vi "Main.vi"() -> ()   [LabVIEW 2018] (continued)
                w3479 = u8 132 items=["I/O (P)"=128, "Input (I)"=129, "Output (Q)"=130, "Bit Memory (M)"=131, "Data (DB)"=132, "Instance Data (DI)"=133, "Local Data (L)"=134, "Predecessor Local Data (VL)"=135] ("寄存器类型")
                w3480 = u16 1 items=["byte", "word", "Dword"] ("数据类型")
                n2689 = local read "上一站号 (301)"() -> (w3472:string)
                n2690 = local read "上一站结果 (301)"() -> (w3471:string)
                n2691 = Decimal String To Number(string=w3472, default (0L)=u32 0 ("默认(0 I32)")) -> (number=w3489:u32)  [unwired: 1 in, 1 out]
                n2692 = call "S7_Write.vi"("TCP"=w3477, "寄存器类型"=w3479, "DB #"=u16 20, "写入地址"=u32 16, "数据类型"=w3480, "写入数据"=w3489, "error in"=w3476) -> ("TCP"=w3488:refnum<k5>, "error out"=w3487:errorcluster)  [unwired: 6 in, 1 out]
                n2693 = Equal?(x=w3471, y="OK") -> (x = y?=w3491:bool)
                n2694 = case shown="假" w3491 {
                  tunnel: [u32 2 ("写入数据") u32 1 ("写入数据")] -> w3492
                  frame False {
                  }
                  frame True {
                  }
                }
                n2695 = local read "扫码请求回复301"() -> (w3470:string)
                n2696 = call "S7_Write.vi"("TCP"=w3488, "寄存器类型"=w3485, "DB #"=u16 20, "写入地址"=u32 18, "数据类型"=w3484, "写入数据"=w3492, "error in"=w3487) -> ("TCP"=w3475:refnum<k5>, "error out"=w3474:errorcluster)  [unwired: 6 in, 1 out]
                n2697 = Decimal String To Number(string=w3470) -> (number=w3473:i32)  [unwired: 2 in, 1 out]
              }
            }
            n2698 = call "S7_Write.vi"("TCP"=w3395, "寄存器类型"=w3413, "DB #"=u16 20, "写入地址"=u32 4, "数据类型"=w3412, "写入数据"=w3393, "error in"=w3394) -> ("TCP"=w3388:refnum<k5>, "error out"=w3387:errorcluster)  [unwired: 6 in, 1 out]
            n2699 = case shown="真" "301数据回复输入" {
              tunnel: [999 w3466] -> w3386
              frame False {
              }
              frame True {
                n2700 = local read "数据保存请求回复301"() -> (w3465:string)
                n2701 = Decimal String To Number(string=w3465) -> (number=w3466:i32)  [unwired: 2 in, 1 out]
              }
            }
            n2702 = call "S7_Write.vi"("TCP"=w3388, "寄存器类型"=w3390, "DB #"=u16 20, "写入地址"=u32 6, "数据类型"=w3389, "写入数据"=w3386, "error in"=w3387) -> ("TCP"=w3385:refnum<k5>, "error out"=w3384:errorcluster)  [unwired: 6 in, 1 out]
            n2703 = case shown="真" "302扫码回复输入" {
              tunnel: [999 w3504] -> w3407
              tunnel: w3385 -> [w3499 w3518]
              tunnel: w3384 -> [w3498 w3517]
              tunnel: [w3499 w3506] -> w3406
              tunnel: [w3498 w3505] -> w3405
              frame False {
              }
              frame True {
                w3512 = u8 132 items=["I/O (P)"=128, "Input (I)"=129, "Output (Q)"=130, "Bit Memory (M)"=131, "Data (DB)"=132, "Instance Data (DI)"=133, "Local Data (L)"=134, "Predecessor Local Data (VL)"=135] ("寄存器类型")
                w3513 = u16 1 items=["byte", "word", "Dword"] ("数据类型")
                w3520 = u8 132 items=["I/O (P)"=128, "Input (I)"=129, "Output (Q)"=130, "Bit Memory (M)"=131, "Data (DB)"=132, "Instance Data (DI)"=133, "Local Data (L)"=134, "Predecessor Local Data (VL)"=135] ("寄存器类型")
                w3519 = u16 1 items=["byte", "word", "Dword"] ("数据类型")
                n2704 = local read "上一站号 (302)"() -> (w3503:string)
                n2705 = Decimal String To Number(string=w3503) -> (number=w3516:i32)  [unwired: 2 in, 1 out]
                n2706 = call "S7_Write.vi"("TCP"=w3518, "寄存器类型"=w3520, "DB #"=u16 20, "写入地址"=u32 20, "数据类型"=w3519, "写入数据"=w3516, "error in"=w3517) -> ("TCP"=w3508:refnum<k5>, "error out"=w3509:errorcluster)  [unwired: 6 in, 1 out]
                n2707 = local read "上一站结果 (302)"() -> (w3502:string)
                n2708 = local read "扫码请求回复302"() -> (w3501:string)
                n2709 = Equal?(x=w3502, y="OK") -> (x = y?=w3515:bool)
                n2710 = case shown="假" w3515 {
                  tunnel: [u32 2 ("写入数据") u32 1 ("写入数据")] -> w3507
                  frame False {
                  }
                  frame True {
                  }
                }
                n2711 = call "S7_Write.vi"("TCP"=w3508, "寄存器类型"=w3512, "DB #"=u16 20, "写入地址"=u32 22, "数据类型"=w3513, "写入数据"=w3507, "error in"=w3509) -> ("TCP"=w3506:refnum<k5>, "error out"=w3505:errorcluster)  [unwired: 6 in, 1 out]
                n2712 = Decimal String To Number(string=w3501) -> (number=w3504:i32)  [unwired: 2 in, 1 out]
              }
            }
            n2713 = call "S7_Write.vi"("TCP"=w3406, "寄存器类型"=w3410, "DB #"=u16 20, "写入地址"=u32 8, "数据类型"=w3411, "写入数据"=w3407, "error in"=w3405) -> ("TCP"=w3399:refnum<k5>, "error out"=w3400:errorcluster)  [unwired: 6 in, 1 out]
            n2714 = case shown="真" "302数据回复输入" {
              tunnel: [999 w3497] -> w3398
              frame False {
              }
              frame True {
                n2715 = local read "数据保存请求回复302"() -> (w3496:string)
                n2716 = Decimal String To Number(string=w3496) -> (number=w3497:i32)  [unwired: 2 in, 1 out]
              }
            }
            n2717 = call "S7_Write.vi"("TCP"=w3399, "寄存器类型"=w3403, "DB #"=u16 20, "写入地址"=u32 10, "数据类型"=w3404, "写入数据"=w3398, "error in"=w3400) -> ("TCP"=w3363:refnum<k5>, "error out"=w3362:errorcluster)  [unwired: 6 in, 1 out]
            n2718 = case shown="真" "303扫码回复输入" {
              tunnel: [999 w3443] -> w3368
              tunnel: w3363 -> [w3438 w3457]
              tunnel: w3362 -> [w3437 w3456]
              tunnel: [w3438 w3445] -> w3369
              tunnel: [w3437 w3444] -> w3370
              frame False {
              }
              frame True {
                w3451 = u8 132 items=["I/O (P)"=128, "Input (I)"=129, "Output (Q)"=130, "Bit Memory (M)"=131, "Data (DB)"=132, "Instance Data (DI)"=133, "Local Data (L)"=134, "Predecessor Local Data (VL)"=135] ("寄存器类型")
                w3452 = u16 1 items=["byte", "word", "Dword"] ("数据类型")
                w3459 = u8 132 items=["I/O (P)"=128, "Input (I)"=129, "Output (Q)"=130, "Bit Memory (M)"=131, "Data (DB)"=132, "Instance Data (DI)"=133, "Local Data (L)"=134, "Predecessor Local Data (VL)"=135] ("寄存器类型")
                w3458 = u16 1 items=["byte", "word", "Dword"] ("数据类型")
                n2719 = local read "上一站号 (303)"() -> (w3442:string)
                n2720 = Decimal String To Number(string=w3442) -> (number=w3455:i32)  [unwired: 2 in, 1 out]
                n2721 = call "S7_Write.vi"("TCP"=w3457, "寄存器类型"=w3459, "DB #"=u16 20, "写入地址"=u32 24, "数据类型"=w3458, "写入数据"=w3455, "error in"=w3456) -> ("TCP"=w3447:refnum<k5>, "error out"=w3448:errorcluster)  [unwired: 6 in, 1 out]
                n2722 = local read "上一站结果 (303)"() -> (w3441:string)
                n2723 = local read "扫码请求回复303"() -> (w3440:string)
                n2724 = Equal?(x=w3441, y="OK") -> (x = y?=w3454:bool)
                n2725 = case shown="假" w3454 {
                  tunnel: [u32 2 ("写入数据") u32 1 ("写入数据")] -> w3446
                  frame False {
                  }
                  frame True {
                  }
                }
                n2726 = call "S7_Write.vi"("TCP"=w3447, "寄存器类型"=w3451, "DB #"=u16 20, "写入地址"=u32 26, "数据类型"=w3452, "写入数据"=w3446, "error in"=w3448) -> ("TCP"=w3445:refnum<k5>, "error out"=w3444:errorcluster)  [unwired: 6 in, 1 out]
                n2727 = Decimal String To Number(string=w3440) -> (number=w3443:i32)  [unwired: 2 in, 1 out]
              }
            }
            n2728 = call "S7_Write.vi"("TCP"=w3369, "寄存器类型"=w3365, "DB #"=u16 20, "写入地址"=u32 12, "数据类型"=w3364, "写入数据"=w3368, "error in"=w3370) -> ("TCP"=w3376:refnum<k5>, "error out"=w3375:errorcluster)  [unwired: 6 in, 1 out]
            n2729 = case shown="真" "303数据回复输入" {
              tunnel: [999 w3436] -> w3377
              frame False {
              }
              frame True {
                n2730 = local read "数据保存请求回复303"() -> (w3435:string)
                n2731 = Decimal String To Number(string=w3435) -> (number=w3436:i32)  [unwired: 2 in, 1 out]
              }
            }
            n2732 = call "S7_Write.vi"("TCP"=w3376, "寄存器类型"=w3372, "DB #"=u16 20, "写入地址"=u32 14, "数据类型"=w3371, "写入数据"=w3377, "error in"=w3375) -> ("TCP"=w3358:refnum<k5>, "error out"=w3359:errorcluster)  [unwired: 6 in, 1 out]
            n2733 = disable-structure shown="启用" {
              disable-tunnel: w3358 -> [w3423 w3427]
              disable-tunnel: [w3423 w3430] -> w3357
              disable-tunnel: w3359 -> [w3424 w3428]
              disable-tunnel: [w3424 w3429] -> w3356
              frame Disabled {
              }
              frame Enabled {
                w3432 = u8 132 items=["I/O (P)"=128, "Input (I)"=129, "Output (Q)"=130, "Bit Memory (M)"=131, "Data (DB)"=132, "Instance Data (DI)"=133, "Local Data (L)"=134, "Predecessor Local Data (VL)"=135] ("寄存器类型")
                w3426 = u16 1 items=["byte", "word", "Dword"] ("数据类型")
                n2734 = local read "产品型号"() -> (w3425:u32)
                n2735 = call "S7_Write.vi"("TCP"=w3427, "寄存器类型"=w3432, "DB #"=u16 20, "写入地址"=u32 174, "数据类型"=w3426, "写入数据"=w3425, "error in"=w3428) -> ("TCP"=w3430:refnum<k5>, "error out"=w3429:errorcluster)  [unwired: 6 in, 1 out]
              }
            }
          }
          frame "错误" {
            n2736 = call "S7_Close.vi"("TCP Connection Ref"=w3529) -> ("error out"=w3530:errorcluster)  [unwired: 10 in]
            n2737 = call <vilib>:"Clear Errors.vi"("error in (no error)"=w3530) -> ()  [unwired: 5 in, 2 out]
          }
          frame "退出" {
            n2738 = call "S7_Close.vi"("TCP Connection Ref"=w3536) -> ("error out"=w3537:errorcluster)  [unwired: 10 in]
            n2739 = call <vilib>:"Clear Errors.vi"("error in (no error)"=w3537) -> ()  [unwired: 5 in, 2 out]
          }
        }
      }
      n2740 = while {
        shift-right: [w925] -> _
        shift-left: errorcluster {"status"=FALSE, "code"=0, "source"=""} ("错误常量") -> [w928]
        shift-right: [w924] -> _
        shift-left: enum16{"初始化", "读", "写", "错误", "退出"}."初始化" -> [w929]
        shift-right: [w926] -> _
        shift-left: _ -> [w923]
        stop <- w922 stop-if-true
        n2741 = local read "退出"() -> (w930:bool)
        n2742 = case shown="假" w930 {
          tunnel: w929 -> [w931 _]
          tunnel: [w932 enum16{"初始化", "读", "写", "错误", "退出"}."退出"] -> w921
          tunnel: w928 -> [w933 _]
          frame False {
            n2743 = case shown="错误" w933 {
              tunnel: [w934 enum16{"初始化", "读", "写", "错误", "退出"}."错误"] -> w932
              tunnel: w931 -> [w934 _]
              frame No Error {
              }
              frame Error {
              }
            }
          }
          frame True {
          }
        }
        n2744 = Wait (ms)(milliseconds to wait=u32 80 ("等待时间（毫秒）")) -> ()  [unwired: 1 out]
        n2745 = case shown="\"读\"" w921 {
          tunnel: [w941 w998 w1142 refnum<k5> refnum ("TCP") refnum<k5> refnum ("TCP")] -> w926
          tunnel: [w942 w997 w1141 errorcluster {"status"=FALSE, "code"=0, "source"=""} ("error out") errorcluster {"status"=FALSE, "code"=0, "source"=""} ("error out")] -> w925
          tunnel: [enum16{"初始化", "读", "写", "错误", "退出"}."读" enum16{"初始化", "读", "写", "错误", "退出"}."写" enum16{"初始化", "读", "写", "错误", "退出"}."读" enum16{"初始化", "读", "写", "错误", "退出"}."初始化" enum16{"初始化", "读", "写", "错误", "退出"}."退出"] -> w924
          tunnel: w923 -> [_ w1034 w1155 w1180 w1187]
          tunnel: [FALSE FALSE FALSE FALSE TRUE] -> w922
          frame "初始化", Default {
            w945 = u16 0 items=["byte", "word", "Dword"] ("数据类型")
            w947 = u8 132 items=["I/O (P)"=128, "Input (I)"=129, "Output (Q)"=130, "Bit Memory (M)"=131, "Data (DB)"=132, "Instance Data (DI)"=133, "Local Data (L)"=134, "Predecessor Local Data (VL)"=135] ("寄存器类型")
            w957 = u8 0 items=["S7-1200.200.200SMART"=0, "S7-300"=2, "S7-400"=3] ("PLC 系列")
            n2746 = call "S7_Open.vi"("IP 地址"="192.168.1.70", "PLC 系列"=w957, "超时（MS）"=100) -> ("TCP"=w944:refnum<k5>, "error out"=w943:errorcluster)  [unwired: 10 in, 1 out]
            n2747 = case shown="错误" w943 {
              tunnel: [FALSE TRUE] -> w953
              frame No Error {
              }
              frame Error {
              }
            }
            n2748 = local write "ST70通讯状态"(w953) -> ()
            n2749 = call "S7_Read.vi"("TCP"=w944, "DB #"=u16 20, "读取长度"=u16 14, "寄存器类型"=w947, "起始地址"=u32 6, "数据类型"=w945, "error in"=w943) -> ("TCP"=w941:refnum<k5>, "数据"=w952:u32[], "error out"=w950:errorcluster)  [unwired: 5 in, 1 out]
            n2750 = To Unsigned Word Integer(number=w952) -> (unsigned 16bit integer=w951:u16[])
            n2751 = call "还原为字符串.vi"("error in (no error)"=w950, "输入数组"=w951) -> ("error out"=w942:errorcluster, "字符串"=w940:string)  [unwired: 8 in]
            n2752 = String To Byte Array(string=w940) -> (unsigned byte array=w939:u8[])
            n2753 = for {
              tunnel: w939 -> [w960] mode=indexing
              tunnel: [w959] -> w938 mode=indexing
              n2754 = Equal?(x=w960, y=u8 32) -> (x = y?=w961:bool)
              n2755 = case shown="真" w961 {
                tunnel: w960 -> [w963 _]
                tunnel: [w963 u8 48] -> w959
                frame False {
                }
                frame True {
                }
              }
            }
            n2756 = Byte Array To String(unsigned byte array=w938) -> (string=w937:string)
            n2757 = local write "70编码"(w937) -> ()
          }
          frame "读" {
            w968 = 15 ("长度")
            w1001 = u16 0 items=["byte", "word", "Dword"] ("数据类型")
            w1003 = u8 132 items=["I/O (P)"=128, "Input (I)"=129, "Output (Q)"=130, "Bit Memory (M)"=131, "Data (DB)"=132, "Instance Data (DI)"=133, "Local Data (L)"=134, "Predecessor Local Data (VL)"=135] ("寄存器类型")
            w1012 = u16 0 items=["byte", "word", "Dword"] ("数据类型")
            w1010 = u8 132 items=["I/O (P)"=128, "Input (I)"=129, "Output (Q)"=130, "Bit Memory (M)"=131, "Data (DB)"=132, "Instance Data (DI)"=133, "Local Data (L)"=134, "Predecessor Local Data (VL)"=135] ("寄存器类型")
            w1023 = 15 ("长度")
            w1035 = u16 0 items=["byte", "word", "Dword"] ("数据类型")
            w1037 = u8 132 items=["I/O (P)"=128, "Input (I)"=129, "Output (Q)"=130, "Bit Memory (M)"=131, "Data (DB)"=132, "Instance Data (DI)"=133, "Local Data (L)"=134, "Predecessor Local Data (VL)"=135] ("寄存器类型")
            n2758 = call "S7_Read.vi"("TCP"=w1034, "DB #"=u16 20, "读取长度"=u16 1, "寄存器类型"=w1037, "起始地址"=u32 0, "数据类型"=w1035) -> ("TCP"=w1030:refnum<k5>, "数据"=w1042:u32[], "读取成功"=w1045:bool, "error out"=w1029:errorcluster)  [unwired: 6 in]
            n2759 = Not(x=w1045) -> (.not. x?=→"ST70通讯状态":bool)
            n2760 = Index Array(array=w1042, index=0 ("索引")) -> (element=w1043:u32)
            n2761 = Number To Boolean Array(number=w1043) -> (Boolean array=w1044:bool[])
            n2762 = Index Array(array=w1044, index=1 ("索引")) -> (element=w967:bool)
            "ST70数据读取" <- w967
            n2763 = call <vilib>:"Boolean Crossing PtByPt.vi"("direction"=enum16{"either", "false-true", "true-false"}."true-false", "input"=w967) -> ()  [unwired: 1 in, 1 out]
            n2764 = case shown="假" w967 {
              frame False {
                n2765 = local write "70数据回复输入"(FALSE ("301数据回复输入")) -> ()
              }
              frame True {
              }
            }
            n2766 = call <vilib>:"Boolean Crossing PtByPt.vi"("direction"=enum16{"either", "false-true", "true-false"}."false-true", "input"=w967) -> ("crossing"=w1028:bool)  [unwired: 1 in]
            n2767 = case shown="真" w1028 {
              tunnel: w1030 -> [w1049 w1085]
              tunnel: w1029 -> [w1048 w1084]
              tunnel: [w1049 w1094] -> w1007
              tunnel: [w1048 w1052] -> w1006
              frame False {
              }
              frame True {
                w1073 = u16 2 items=["byte", "word", "Dword"] ("数据类型")
                w1075 = u8 132 items=["I/O (P)"=128, "Input (I)"=129, "Output (Q)"=130, "Bit Memory (M)"=131, "Data (DB)"=132, "Instance Data (DI)"=133, "Local Data (L)"=134, "Predecessor Local Data (VL)"=135] ("寄存器类型")
                w1086 = u16 0 items=["byte", "word", "Dword"] ("数据类型")
                w1088 = u8 132 items=["I/O (P)"=128, "Input (I)"=129, "Output (Q)"=130, "Bit Memory (M)"=131, "Data (DB)"=132, "Instance Data (DI)"=133, "Local Data (L)"=134, "Predecessor Local Data (VL)"=135] ("寄存器类型")
                w1099 = u16 2 items=["byte", "word", "Dword"] ("数据类型")
                w1097 = u8 132 items=["I/O (P)"=128, "Input (I)"=129, "Output (Q)"=130, "Bit Memory (M)"=131, "Data (DB)"=132, "Instance Data (DI)"=133, "Local Data (L)"=134, "Predecessor Local Data (VL)"=135] ("寄存器类型")
                w1100 = u16 1 items=["byte", "word", "Dword"] ("数据类型")
                w1102 = u8 132 items=["I/O (P)"=128, "Input (I)"=129, "Output (Q)"=130, "Bit Memory (M)"=131, "Data (DB)"=132, "Instance Data (DI)"=133, "Local Data (L)"=134, "Predecessor Local Data (VL)"=135] ("寄存器类型")
                n2768 = call "S7_Read.vi"("TCP"=w1085, "DB #"=u16 20, "读取长度"=u16 14, "寄存器类型"=w1088, "起始地址"=u32 6, "数据类型"=w1086, "error in"=w1084) -> ("TCP"=w1082:refnum<k5>, "数据"=w1093:u32[], "error out"=w1091:errorcluster)  [unwired: 5 in, 1 out]
                n2769 = To Unsigned Word Integer(number=w1093) -> (unsigned 16bit integer=w1092:u16[])
                n2770 = call "还原为字符串.vi"("error in (no error)"=w1091, "输入数组"=w1092) -> ("error out"=w1083:errorcluster, "字符串"=w1053:string)  [unwired: 8 in]
                n2771 = String To Byte Array(string=w1053) -> (unsigned byte array=w1055:u8[])
                n2772 = for {
                  tunnel: w1055 -> [w1133] mode=indexing
                  tunnel: [w1132] -> w1054 mode=indexing
                  n2773 = Equal?(x=w1133, y=u8 32) -> (x = y?=w1134:bool)
                  n2774 = case shown="真" w1134 {
                    tunnel: w1133 -> [w1136 _]
                    tunnel: [w1136 u8 48] -> w1132
                    frame False {
                    }
                    frame True {
                    }
                  }
                }
                n2775 = call "S7_Read.vi"("TCP"=w1082, "DB #"=u16 20, "读取长度"=u16 12, "寄存器类型"=w1097, "起始地址"=u32 20, "数据类型"=w1099, "error in"=w1083) -> ("TCP"=w1071:refnum<k5>, "数据"=w1070:u32[], "error out"=w1072:errorcluster)  [unwired: 5 in, 1 out]
                n2776 = Byte Array To String(unsigned byte array=w1054) -> (string=w1050:string)
                "70编码" <- w1050
                n2777 = Divide(x=w1070, y=u32[] [100, 100, 100, 100, 100, 100, 100, 100, 100, 100, 100, 100]) -> (x/y=w1068:dbl[])
                n2778 = Number To Fractional String(number=w1068, precision (6)=i16 2 ("精度(6)")) -> (F-format string=w1067:string[])  [unwired: 2 in]
                n2779 = call "S7_Read.vi"("TCP"=w1071, "DB #"=u16 20, "读取长度"=u16 6, "寄存器类型"=w1075, "起始地址"=u32 152, "数据类型"=w1073, "error in"=w1072) -> ("TCP"=w1066:refnum<k5>, "数据"=w1062:u32[], "error out"=w1065:errorcluster)  [unwired: 5 in, 1 out]
                n2780 = Divide(x=w1062, y=u32[] [100, 100, 100, 100, 100, 100]) -> (x/y=w1064:dbl[])
                n2781 = Number To Fractional String(number=w1064, precision (6)=i16 2 ("精度(6)")) -> (F-format string=w1059:string[])  [unwired: 2 in]
                n2782 = call "S7_Read.vi"("TCP"=w1066, "DB #"=u16 20, "读取长度"=u16 1, "寄存器类型"=w1102, "起始地址"=u32 68, "数据类型"=w1100, "error in"=w1065) -> ("TCP"=w1094:refnum<k5>, "数据"=w1110:u32[], "error out"=w1056:errorcluster)  [unwired: 5 in, 1 out]
                n2783 = Index Array(array=w1110) -> (element=w1112:u32)  [unwired: 1 in]
                n2784 = local read "ST70_Housing_5025351"() -> (w1057:string)
                n2785 = local read "ST70_Bushing_5025400"() -> (w1058:string)
                n2786 = Equal?(x=w1112, y=u32 1) -> (x = y?=w1111:bool)
                n2787 = case shown="真" w1111 {
                  tunnel: ["NG" "OK"] -> w1079
                  frame False {
                  }
                  frame True {
                  }
                }
                n2788 = Format Date/Time String(time format string (%c)="%Y-%m-%d" ("时间格式字符串(%c)")) -> (date/time string=w1080:string)  [unwired: 2 in]
                n2789 = Get Date/Time String(want seconds? (F)=TRUE ("需要秒？(F)")) -> (time string=w1081:string)  [unwired: 2 in, 1 out]
                n2790 = Insert Into Array(array=string[] [] ("数组"), index=0 ("索引"), new element #1=w1050, new element #2="70" ("新元素/子数组"), new element #3=w1079, new element #4=w1080, new element #5=w1081, new element #6=w1079, new element #7=w1067, new element #8=w1059, new element #9=w1058, new element #10=w1057) -> (w1051:string[])
                n2791 = stacked-sequence {
                  seq-local: [_ w1114 _] -> [_ _ w1118]
                  tunnel: w1056 -> [_ _ w1120]
                  tunnel: [_ _ w1119] -> w1052
                  tunnel: w1051 -> [w1113 _ _]
                  tunnel: w1050 -> [_ w1117 _]
                  frame #0 {
                    "70数据" <- w1113
                  }
                  frame #1 {
                    n2792 = call <vilib>:"Trim Whitespace.vi"("string"=w1117) -> ("trimmed string"=w1116:string)  [unwired: 1 in]
                    n2793 = Not Equal?(x=w1116, y="") -> (x != y?=w1114:bool)
                  }
                  frame #2 {
                    n2794 = case shown="假" w1118 {
                      tunnel: w1120 -> [w1123 w1127]
                      tunnel: [w1123 w1124] -> w1119
                      frame False {
                        n2795 = local write "70数据回复输入"(TRUE ("70数据回复输入")) -> ()
                        n2796 = local write "数据保存请求回复70"("2" ("数据保存请求回复70")) -> ()
                      }
                      frame True {
                        n2797 = property on="ST70数据读取（事件）" class="Bool (严格)"(error in=w1127, "Val(Sgnl)"=TRUE ("值(信号)")) -> (error out=w1125:errorcluster)  [unwired: 1 in, 1 out]
                        n2798 = disable-structure shown="禁用" {
                          disable-tunnel: w1125 -> [w1129 w1131]
                          disable-tunnel: [w1128 w1131] -> w1124
                          frame Disabled {
                            n2799 = property on="ST70画曲线" class="Bool (严格)"(error in=w1129, "Val(Sgnl)"=TRUE ("值(信号)")) -> (error out=w1128:errorcluster)  [unwired: 1 in, 1 out]
                          }
                          frame Enabled {
                          }
                        }
                      }
                    }
                  }
                }
              }
            }
            n2800 = call "S7_Read.vi"("TCP"=w1007, "DB #"=u16 20, "读取长度"=u16 30, "寄存器类型"=w1010, "起始地址"=u32 72, "数据类型"=w1012, "error in"=w1006) -> ("TCP"=w1000:refnum<k5>, "数据"=w996:u32[], "error out"=w999:errorcluster)  [unwired: 5 in, 1 out]
            n2801 = Delete From Array(array=w996, length=w1023, index=2 ("索引")) -> (deleted portion=w1016:u32[])  [unwired: 1 out]
            n2802 = Delete From Array(array=w996, length=w1023, index=17 ("索引")) -> (deleted portion=w1020:u32[])  [unwired: 1 out]
            n2803 = To Unsigned Word Integer(number=w1016) -> (unsigned 16bit integer=w1013:u16[])
            n2804 = To Unsigned Word Integer(number=w1020) -> (unsigned 16bit integer=w1019:u16[])
            n2805 = call "还原为字符串.vi"("输入数组"=w1013) -> ("字符串"=w1015:string)  [unwired: 9 in, 1 out]
            n2806 = call "还原为字符串.vi"("输入数组"=w1019) -> ("字符串"=w1017:string)  [unwired: 9 in, 1 out]
            n2807 = Match Pattern(string=w1015, regular expression="\r" ("正则表达式")) -> (before substring=w1014:string)  [unwired: 1 in, 3 out]
            n2808 = Match Pattern(string=w1017, regular expression="\r" ("正则表达式")) -> (before substring=w1018:string)  [unwired: 1 in, 3 out]
            n2809 = Match Pattern(string=w1014, regular expression="\u0000" ("正则表达式")) -> (before substring=→"ST70_Housing_5025351":string)  [unwired: 1 in, 3 out]
            n2810 = Match Pattern(string=w1018, regular expression="\u0000" ("正则表达式")) -> (before substring=→"ST70_Bushing_5025400":string)  [unwired: 1 in, 3 out]
            n2811 = call "S7_Read.vi"("TCP"=w1000, "DB #"=u16 20, "读取长度"=u16 30, "寄存器类型"=w1003, "起始地址"=u32 104, "数据类型"=w1001, "error in"=w999) -> ("TCP"=w998:refnum<k5>, "数据"=w969:u32[], "error out"=w997:errorcluster)  [unwired: 5 in, 1 out]
            n2812 = Delete From Array(array=w969, length=w968, index=2 ("索引")) -> (deleted portion=w988:u32[])  [unwired: 1 out]
            n2813 = Delete From Array(array=w969, length=w968, index=18 ("索引")) -> (deleted portion=w984:u32[])  [unwired: 1 out]
            n2814 = Delete From Array(array=w969, length=w968, index=35 ("索引")) -> (deleted portion=w974:u32[])  [unwired: 1 out]
            n2815 = To Unsigned Word Integer(number=w988) -> (unsigned 16bit integer=w991:u16[])
            n2816 = To Unsigned Word Integer(number=w984) -> (unsigned 16bit integer=w985:u16[])
            n2817 = To Unsigned Word Integer(number=w974) -> (unsigned 16bit integer=w973:u16[])
            n2818 = call "还原为字符串.vi"("输入数组"=w991) -> ("字符串"=w989:string)  [unwired: 9 in, 1 out]
            n2819 = call "还原为字符串.vi"("输入数组"=w985) -> ("字符串"=w987:string)  [unwired: 9 in, 1 out]
            n2820 = call "还原为字符串.vi"("输入数组"=w973) -> ("字符串"=w971:string)  [unwired: 9 in, 1 out]
            n2821 = Match Pattern(string=w989, regular expression="\r" ("正则表达式")) -> (before substring=w990:string)  [unwired: 1 in, 3 out]
            n2822 = Match Pattern(string=w987, regular expression="\r" ("正则表达式")) -> (before substring=w986:string)  [unwired: 1 in, 3 out]
            n2823 = Match Pattern(string=w971, regular expression="\r" ("正则表达式")) -> (before substring=w972:string)  [unwired: 1 in, 3 out]
            n2824 = Match Pattern(string=w990, regular expression="\u0000" ("正则表达式")) -> (before substring=→"ST80_Flat_sael_5020064":string)  [unwired: 1 in, 3 out]
            n2825 = Match Pattern(string=w986, regular expression="\u0000" ("正则表达式")) -> (before substring=→"ST80_Spring_5024883":string)  [unwired: 1 in, 3 out]
            n2826 = Match Pattern(string=w972, regular expression="\u0000" ("正则表达式")) -> (before substring=→"ST80_Spring_plate_5025473":string)  [unwired: 1 in, 3 out]
          }
          frame "写" {
            w1152 = u8 132 items=["I/O (P)"=128, "Input (I)"=129, "Output (Q)"=130, "Bit Memory (M)"=131, "Data (DB)"=132, "Instance Data (DI)"=133, "Local Data (L)"=134, "Predecessor Local Data (VL)"=135] ("寄存器类型")
            w1151 = u16 1 items=["byte", "word", "Dword"] ("数据类型")
            w1159 = u8 132 items=["I/O (P)"=128, "Input (I)"=129, "Output (Q)"=130, "Bit Memory (M)"=131, "Data (DB)"=132, "Instance Data (DI)"=133, "Local Data (L)"=134, "Predecessor Local Data (VL)"=135] ("寄存器类型")
            w1156 = u16 1 items=["byte", "word", "Dword"] ("数据类型")
            n2827 = local read "70看门狗"() -> (w1149:i32)
            n2828 = case shown="0" w1149 {
              tunnel: [0 ("y") 1 ("y")] -> w1148
              frame 1, Default {
              }
              frame 0 {
              }
            }
            "70看门狗" <- w1148
            n2829 = call "S7_Write.vi"("TCP"=w1155, "寄存器类型"=w1159, "DB #"=u16 20, "写入地址"=u32 2, "数据类型"=w1156, "写入数据"=w1148) -> ("TCP"=w1146:refnum<k5>, "error out"=w1145:errorcluster)  [unwired: 7 in, 1 out]
            n2830 = case shown="真" "70数据回复输入" {
              tunnel: [999 w1175] -> w1150
              frame False {
              }
              frame True {
                n2831 = local read "数据保存请求回复70"() -> (w1174:string)
                n2832 = Decimal String To Number(string=w1174) -> (number=w1175:i32)  [unwired: 2 in, 1 out]
              }
            }
            n2833 = call "S7_Write.vi"("TCP"=w1146, "寄存器类型"=w1152, "DB #"=u16 20, "写入地址"=u32 4, "数据类型"=w1151, "写入数据"=w1150, "error in"=w1145) -> ("TCP"=w1144:refnum<k5>, "error out"=w1143:errorcluster)  [unwired: 6 in, 1 out]
            n2834 = disable-structure shown="启用" {
              disable-tunnel: w1144 -> [w1162 w1166]
              disable-tunnel: [w1162 w1169] -> w1142
              disable-tunnel: w1143 -> [w1163 w1167]
              disable-tunnel: [w1163 w1168] -> w1141
              frame Disabled {
              }
              frame Enabled {
                w1171 = u8 132 items=["I/O (P)"=128, "Input (I)"=129, "Output (Q)"=130, "Bit Memory (M)"=131, "Data (DB)"=132, "Instance Data (DI)"=133, "Local Data (L)"=134, "Predecessor Local Data (VL)"=135] ("寄存器类型")
                w1165 = u16 1 items=["byte", "word", "Dword"] ("数据类型")
                n2835 = local read "产品型号"() -> (w1164:u32)
                n2836 = call "S7_Write.vi"("TCP"=w1166, "寄存器类型"=w1171, "DB #"=u16 20, "写入地址"=u32 176, "数据类型"=w1165, "写入数据"=w1164, "error in"=w1167) -> ("TCP"=w1169:refnum<k5>, "error out"=w1168:errorcluster)  [unwired: 6 in, 1 out]
              }
            }
          }
          frame "错误" {
            n2837 = call "S7_Close.vi"("TCP Connection Ref"=w1180) -> ("error out"=w1181:errorcluster)  [unwired: 10 in]
            n2838 = call <vilib>:"Clear Errors.vi"("error in (no error)"=w1181) -> ()  [unwired: 5 in, 2 out]
          }
          frame "退出" {
            n2839 = call "S7_Close.vi"("TCP Connection Ref"=w1187) -> ("error out"=w1188:errorcluster)  [unwired: 10 in]
            n2840 = call <vilib>:"Clear Errors.vi"("error in (no error)"=w1188) -> ()  [unwired: 5 in, 2 out]
          }
        }
      }
      n2841 = while {
        shift-right: [w1752] -> _
        shift-left: errorcluster {"status"=FALSE, "code"=0, "source"=""} ("错误常量") -> [w1755]
        shift-right: [w1751] -> _
        shift-left: enum16{"初始化", "读", "写", "错误", "退出"}."初始化" -> [w1756]
        shift-right: [w1753] -> _
        shift-left: _ -> [w1750]
        stop <- w1749 stop-if-true
        n2842 = local read "退出"() -> (w1757:bool)
        n2843 = case shown="假" w1757 {
          tunnel: w1756 -> [w1758 _]
          tunnel: [w1759 enum16{"初始化", "读", "写", "错误", "退出"}."退出"] -> w1748
          tunnel: w1755 -> [w1760 _]
          frame False {
            n2844 = case shown="错误" w1760 {
              tunnel: [w1761 enum16{"初始化", "读", "写", "错误", "退出"}."错误"] -> w1759
              tunnel: w1758 -> [w1761 _]
              frame No Error {
              }
              frame Error {
              }
            }
          }
          frame True {
          }
        }
        n2845 = Wait (ms)(milliseconds to wait=u32 80 ("等待时间（毫秒）")) -> ()  [unwired: 1 out]
        n2846 = case shown="\"读\"" w1748 {
          tunnel: [w1766 w1823 w2388 refnum<k5> refnum ("TCP") refnum<k5> refnum ("TCP")] -> w1753
          tunnel: [w1764 w1822 w2386 errorcluster {"status"=FALSE, "code"=0, "source"=""} ("error out") errorcluster {"status"=FALSE, "code"=0, "source"=""} ("error out")] -> w1752
          tunnel: [enum16{"初始化", "读", "写", "错误", "退出"}."读" enum16{"初始化", "读", "写", "错误", "退出"}."写" enum16{"初始化", "读", "写", "错误", "退出"}."读" enum16{"初始化", "读", "写", "错误", "退出"}."初始化" enum16{"初始化", "读", "写", "错误", "退出"}."退出"] -> w1751
          tunnel: w1750 -> [_ w1870 w2464 w2607 w2614]
          tunnel: [FALSE FALSE FALSE FALSE TRUE] -> w1749
          frame "初始化", Default {
            w1792 = u16 0 items=["byte", "word", "Dword"] ("数据类型")
            w1790 = u8 132 items=["I/O (P)"=128, "Input (I)"=129, "Output (Q)"=130, "Bit Memory (M)"=131, "Data (DB)"=132, "Instance Data (DI)"=133, "Local Data (L)"=134, "Predecessor Local Data (VL)"=135] ("寄存器类型")
            w1776 = u16 0 items=["byte", "word", "Dword"] ("数据类型")
            w1778 = u8 132 items=["I/O (P)"=128, "Input (I)"=129, "Output (Q)"=130, "Bit Memory (M)"=131, "Data (DB)"=132, "Instance Data (DI)"=133, "Local Data (L)"=134, "Predecessor Local Data (VL)"=135] ("寄存器类型")
            w1775 = u16 0 items=["byte", "word", "Dword"] ("数据类型")
            w1773 = u8 132 items=["I/O (P)"=128, "Input (I)"=129, "Output (Q)"=130, "Bit Memory (M)"=131, "Data (DB)"=132, "Instance Data (DI)"=133, "Local Data (L)"=134, "Predecessor Local Data (VL)"=135] ("寄存器类型")
            w1801 = u16 0 items=["byte", "word", "Dword"] ("数据类型")
            w1803 = u8 132 items=["I/O (P)"=128, "Input (I)"=129, "Output (Q)"=130, "Bit Memory (M)"=131, "Data (DB)"=132, "Instance Data (DI)"=133, "Local Data (L)"=134, "Predecessor Local Data (VL)"=135] ("寄存器类型")
            w1814 = u8 0 items=["S7-1200.200.200SMART"=0, "S7-300"=2, "S7-400"=3] ("PLC 系列")
            n2847 = call "S7_Open.vi"("IP 地址"="192.168.1.50", "PLC 系列"=w1814, "超时（MS）"=100) -> ("TCP"=w1800:refnum<k5>, "error out"=w1799:errorcluster)  [unwired: 10 in, 1 out]
            n2848 = call "S7_Read.vi"("TCP"=w1800, "DB #"=u16 20, "读取长度"=u16 13, "寄存器类型"=w1803, "起始地址"=u32 82, "数据类型"=w1801, "error in"=w1799) -> ("TCP"=w1767:refnum<k5>, "数据"=w1806:u32[], "error out"=w1808:errorcluster)  [unwired: 5 in, 1 out]
            n2849 = To Unsigned Word Integer(number=w1806) -> (unsigned 16bit integer=w1807:u16[])
            n2850 = call "还原为字符串.vi"("error in (no error)"=w1808, "输入数组"=w1807) -> ("error out"=w1765:errorcluster, "字符串"=w1809:string)  [unwired: 8 in]
            n2851 = local write "504二维码"(w1809) -> ()
            n2852 = case shown="错误" w1765 {
              tunnel: [FALSE TRUE] -> w1810
              frame No Error {
              }
              frame Error {
              }
            }
            n2853 = local write "ST50通讯状态"(w1810) -> ()
            n2854 = call "S7_Read.vi"("TCP"=w1767, "DB #"=u16 20, "读取长度"=u16 13, "寄存器类型"=w1773, "起始地址"=u32 38, "数据类型"=w1775, "error in"=w1765) -> ("TCP"=w1797:refnum<k5>, "数据"=w1770:u32[], "error out"=w1768:errorcluster)  [unwired: 5 in, 1 out]
            n2855 = To Unsigned Word Integer(number=w1770) -> (unsigned 16bit integer=w1769:u16[])
            n2856 = call "还原为字符串.vi"("error in (no error)"=w1768, "输入数组"=w1769) -> ("error out"=w1798:errorcluster, "字符串"=w1796:string)  [unwired: 8 in]
            n2857 = local write "501二维码"(w1796) -> ()
            n2858 = call "S7_Read.vi"("TCP"=w1797, "DB #"=u16 20, "读取长度"=u16 13, "寄存器类型"=w1778, "起始地址"=u32 60, "数据类型"=w1776, "error in"=w1798) -> ("TCP"=w1794:refnum<k5>, "数据"=w1781:u32[], "error out"=w1783:errorcluster)  [unwired: 5 in, 1 out]
            n2859 = To Unsigned Word Integer(number=w1781) -> (unsigned 16bit integer=w1782:u16[])
            n2860 = call "还原为字符串.vi"("error in (no error)"=w1783, "输入数组"=w1782) -> ("error out"=w1795:errorcluster, "字符串"=w1793:string)  [unwired: 8 in]
            n2861 = local write "502二维码"(w1793) -> ()
            n2862 = call "S7_Read.vi"("TCP"=w1794, "DB #"=u16 20, "读取长度"=u16 13, "寄存器类型"=w1790, "起始地址"=u32 82, "数据类型"=w1792, "error in"=w1795) -> ("TCP"=w1766:refnum<k5>, "数据"=w1787:u32[], "error out"=w1785:errorcluster)  [unwired: 5 in, 1 out]
            n2863 = To Unsigned Word Integer(number=w1787) -> (unsigned 16bit integer=w1786:u16[])
            n2864 = call "还原为字符串.vi"("error in (no error)"=w1785, "输入数组"=w1786) -> ("error out"=w1764:errorcluster, "字符串"=w1784:string)  [unwired: 8 in]
            n2865 = local write "503二维码"(w1784) -> ()
          }
          frame "读" {
            w1871 = u16 0 items=["byte", "word", "Dword"] ("数据类型")
            w1873 = u8 132 items=["I/O (P)"=128, "Input (I)"=129, "Output (Q)"=130, "Bit Memory (M)"=131, "Data (DB)"=132, "Instance Data (DI)"=133, "Local Data (L)"=134, "Predecessor Local Data (VL)"=135] ("寄存器类型")
            n2866 = call "S7_Read.vi"("TCP"=w1870, "DB #"=u16 20, "读取长度"=u16 1, "寄存器类型"=w1873, "起始地址"=u32 0, "数据类型"=w1871) -> ("TCP"=w1868:refnum<k5>, "数据"=w1878:u32[], "读取成功"=w1881:bool, "error out"=w1867:errorcluster)  [unwired: 6 in]
            n2867 = Index Array(array=w1878, index=0 ("索引")) -> (element=w1879:u32)
            n2868 = Not(x=w1881) -> (.not. x?=→"ST50通讯状态":bool)
            n2869 = Number To Boolean Array(number=w1879) -> (Boolean array=w1880:bool[])
            n2870 = Index Array(array=w1880, index #1=0 ("索引")) -> (element #1=w1849:bool, element #2=w1840:bool, element #3=w1839:bool, element #4=w1836:bool, element #5=w1835:bool, element #6=w1832:bool, element #7=w1819:bool, element #8=w1818:bool)  [unwired: 7 in]
            "ST501扫码请求" <- w1849
            "ST501数据读取" <- w1840
            "ST502扫码请求" <- w1839
            "ST502数据读取" <- w1836
            "ST503扫码请求" <- w1835
            "ST503数据读取" <- w1832
            "ST504扫码请求" <- w1819
            "ST504数据读取" <- w1818
            n2871 = disable-structure shown="启用" {
              disable-tunnel: [w1893 w1895] -> w1851
              disable-tunnel: w1849 -> [w1892 w1895]
              frame Disabled {
                n2872 = call <vilib>:"Boolean Crossing PtByPt.vi"("direction"=enum16{"either", "false-true", "true-false"}."true-false", "input"=w1892) -> ("crossing"=w1893:bool)  [unwired: 1 in]
              }
              frame Enabled {
              }
            }
            n2873 = call <vilib>:"Boolean Crossing PtByPt.vi"("direction"=enum16{"either", "false-true", "true-false"}."false-true", "input"=w1849) -> ("crossing"=w1866:bool)  [unwired: 1 in]
            n2874 = case shown="真" w1866 {
              tunnel: w1868 -> [w2367 w2372]
              tunnel: w1867 -> [w2366 w2373]
              tunnel: [w2367 w2371] -> w1865
              tunnel: [w2366 w2370] -> w1864
              frame False {
              }
              frame True {
                w2381 = u16 0 items=["byte", "word", "Dword"] ("数据类型")
                w2379 = u8 132 items=["I/O (P)"=128, "Input (I)"=129, "Output (Q)"=130, "Bit Memory (M)"=131, "Data (DB)"=132, "Instance Data (DI)"=133, "Local Data (L)"=134, "Predecessor Local Data (VL)"=135] ("寄存器类型")
                n2875 = call "S7_Read.vi"("TCP"=w2372, "DB #"=u16 20, "读取长度"=u16 13, "寄存器类型"=w2379, "起始地址"=u32 38, "数据类型"=w2381, "error in"=w2373) -> ("TCP"=w2371:refnum<k5>, "数据"=w2376:u32[], "error out"=w2374:errorcluster)  [unwired: 5 in, 1 out]
                n2876 = To Unsigned Word Integer(number=w2376) -> (unsigned 16bit integer=w2375:u16[])
                n2877 = call "还原为字符串.vi"("error in (no error)"=w2374, "输入数组"=w2375) -> ("error out"=w2369:errorcluster, "字符串"=w2368:string)  [unwired: 8 in]
                n2878 = stacked-sequence {
                  tunnel: [_ w2385] -> w2370
                  tunnel: w2369 -> [_ w2384]
                  tunnel: w2368 -> [w2382 _]
                  frame #0 {
                    "501二维码" <- w2382
                  }
                  frame #1 {
                    n2879 = property on="ST501扫码请求（事件）" class="Bool (严格)"(error in=w2384, "Val(Sgnl)"=TRUE ("值(信号)")) -> (error out=w2385:errorcluster)  [unwired: 1 in, 1 out]
                  }
                }
              }
            }
            n2880 = case shown="假" w1851 {
              frame False {
                n2881 = local write "501扫码回复输入"(FALSE ("301扫码回复输入")) -> ()
              }
              frame True {
              }
            }
            n2882 = disable-structure shown="启用" {
              disable-tunnel: [w1898 w1899] -> w1821
              disable-tunnel: w1819 -> [w1896 w1899]
              frame Disabled {
                n2883 = call <vilib>:"Boolean Crossing PtByPt.vi"("direction"=enum16{"either", "false-true", "true-false"}."true-false", "input"=w1896) -> ("crossing"=w1898:bool)  [unwired: 1 in]
              }
              frame Enabled {
              }
            }
            n2884 = disable-structure shown="启用" {
              disable-tunnel: [w1913 w1915] -> w1860
              disable-tunnel: w1840 -> [w1912 w1915]
              frame Disabled {
                n2885 = call <vilib>:"Boolean Crossing PtByPt.vi"("direction"=enum16{"either", "false-true", "true-false"}."true-false", "input"=w1912) -> ("crossing"=w1913:bool)  [unwired: 1 in]
              }
              frame Enabled {
              }
            }
            n2886 = call <vilib>:"Boolean Crossing PtByPt.vi"("direction"=enum16{"either", "false-true", "true-false"}."false-true", "input"=w1840) -> ("crossing"=w1862:bool)  [unwired: 1 in]
            n2887 = case shown="真" w1862 {
              tunnel: [w2310 w2325] -> w1858
              tunnel: [w2309 w2312] -> w1857
              tunnel: w1864 -> [w2309 w2326]
              tunnel: w1865 -> [w2310 w2327]
              frame False {
              }
              frame True {
                w2341 = u16 1 items=["byte", "word", "Dword"] ("数据类型")
                w2343 = u8 132 items=["I/O (P)"=128, "Input (I)"=129, "Output (Q)"=130, "Bit Memory (M)"=131, "Data (DB)"=132, "Instance Data (DI)"=133, "Local Data (L)"=134, "Predecessor Local Data (VL)"=135] ("寄存器类型")
                w2336 = u16 1 items=["byte", "word", "Dword"] ("数据类型")
                w2338 = u8 132 items=["I/O (P)"=128, "Input (I)"=129, "Output (Q)"=130, "Bit Memory (M)"=131, "Data (DB)"=132, "Instance Data (DI)"=133, "Local Data (L)"=134, "Predecessor Local Data (VL)"=135] ("寄存器类型")
                w2331 = u16 0 items=["byte", "word", "Dword"] ("数据类型")
                w2333 = u8 132 items=["I/O (P)"=128, "Input (I)"=129, "Output (Q)"=130, "Bit Memory (M)"=131, "Data (DB)"=132, "Instance Data (DI)"=133, "Local Data (L)"=134, "Predecessor Local Data (VL)"=135] ("寄存器类型")
                n2888 = call "S7_Read.vi"("TCP"=w2327, "DB #"=u16 20, "读取长度"=u16 1, "寄存器类型"=w2333, "起始地址"=u32 1, "数据类型"=w2331, "error in"=w2326) -> ("TCP"=w2349:refnum<k5>, "数据"=w2318:u32[], "error out"=w2350:errorcluster)  [unwired: 5 in, 1 out]
                n2889 = Index Array(array=w2318, index=0 ("索引")) -> (element=w2321:u32)
                n2890 = Number To Boolean Array(number=w2321) -> (Boolean array=w2322:bool[])
                n2891 = Index Array(array=w2322, index=1 ("索引")) -> (element=w2317:bool)
                n2892 = case shown="真" w2317 {
                  tunnel: ["F" "T"] -> w2314
                  frame False {
                  }
                  frame True {
                  }
                }
                n2893 = call "S7_Read.vi"("TCP"=w2349, "DB #"=u16 20, "读取长度"=u16 1, "寄存器类型"=w2338, "起始地址"=u32 124, "数据类型"=w2336, "error in"=w2350) -> ("TCP"=w2351:refnum<k5>, "数据"=w2353:u32[], "error out"=w2352:errorcluster)  [unwired: 5 in, 1 out]
                n2894 = Index Array(array=w2353) -> (element=w2355:u32)  [unwired: 1 in]
                n2895 = Equal?(x=w2355, y=u32 1) -> (x = y?=w2354:bool)
                n2896 = case shown="真" w2354 {
                  tunnel: ["NG" "OK"] -> w2316
                  frame False {
                  }
                  frame True {
                  }
                }
                n2897 = call "S7_Read.vi"("TCP"=w2351, "DB #"=u16 20, "读取长度"=u16 1, "寄存器类型"=w2343, "起始地址"=u32 132, "数据类型"=w2341, "error in"=w2352) -> ("TCP"=w2325:refnum<k5>, "数据"=w2324:u32[], "error out"=w2313:errorcluster)  [unwired: 5 in, 1 out]
                n2898 = Index Array(array=w2324) -> (element=w2323:u32)  [unwired: 1 in]
                n2899 = Number To Decimal String(number=w2323) -> (decimal integer string=w2315:string)  [unwired: 1 in]
                n2900 = Format Date/Time String(time format string (%c)="%Y-%m-%d" ("时间格式字符串(%c)")) -> (date/time string=w2356:string)  [unwired: 2 in]
                n2901 = Get Date/Time String(want seconds? (F)=TRUE ("需要秒？(F)")) -> (time string=w2357:string)  [unwired: 2 in, 1 out]
                n2902 = Insert Into Array(array=string[] [] ("数组"), index=0 ("索引"), new element #1="501" ("新元素/子数组"), new element #2=w2316, new element #3=w2356, new element #4=w2357, new element #5=w2316, new element #6=w2315, new element #7=w2314) -> (w2311:string[])
                n2903 = stacked-sequence {
                  tunnel: w2313 -> [_ w2361]
                  tunnel: [_ w2360] -> w2312
                  tunnel: w2311 -> [w2358 _]
                  frame #0 {
                    "501data" <- w2358
                  }
                  frame #1 {
                    n2904 = property on="ST501数据读取（事件）" class="Bool (严格)"(error in=w2361, "Val(Sgnl)"=TRUE ("值(信号)")) -> (error out=w2360:errorcluster)  [unwired: 1 in, 1 out]
                  }
                }
              }
            }
            n2905 = case shown="假" w1821 {
              frame False {
                n2906 = local write "504扫码回复输入"(FALSE ("504扫码回复输入")) -> ()
              }
              frame True {
              }
            }
            n2907 = case shown="假" w1860 {
              frame False {
                n2908 = local write "501数据回复输入"(FALSE ("301数据回复输入")) -> ()
              }
              frame True {
              }
            }
            n2909 = disable-structure shown="启用" {
              disable-tunnel: [w1890 w1891] -> w1859
              disable-tunnel: w1839 -> [w1888 w1891]
              frame Disabled {
                n2910 = call <vilib>:"Boolean Crossing PtByPt.vi"("direction"=enum16{"either", "false-true", "true-false"}."true-false", "input"=w1888) -> ("crossing"=w1890:bool)  [unwired: 1 in]
              }
              frame Enabled {
              }
            }
            n2911 = disable-structure shown="启用" {
              disable-tunnel: [w1901 w1903] -> w1820
              disable-tunnel: w1818 -> [w1900 w1903]
              frame Disabled {
                n2912 = call <vilib>:"Boolean Crossing PtByPt.vi"("direction"=enum16{"either", "false-true", "true-false"}."true-false", "input"=w1900) -> ("crossing"=w1901:bool)  [unwired: 1 in]
              }
              frame Enabled {
              }
            }
            n2913 = case shown="假" w1859 {
              frame False {
                n2914 = local write "502扫码回复输入"(FALSE ("302扫码回复输入")) -> ()
              }
              frame True {
              }
            }
            n2915 = case shown="假" w1820 {
              frame False {
                n2916 = local write "504数据回复输入"(FALSE ("504数据回复输入")) -> ()
              }
              frame True {
              }
            }
            n2917 = disable-structure shown="启用" {
              disable-tunnel: [w1909 w1911] -> w1838
              disable-tunnel: w1836 -> [w1908 w1911]
              frame Disabled {
                n2918 = call <vilib>:"Boolean Crossing PtByPt.vi"("direction"=enum16{"either", "false-true", "true-false"}."true-false", "input"=w1908) -> ("crossing"=w1909:bool)  [unwired: 1 in]
              }
              frame Enabled {
              }
            }
            n2919 = case shown="假" w1838 {
              frame False {
                n2920 = local write "502数据回复输入"(FALSE ("302数据回复输入")) -> ()
              }
              frame True {
              }
            }
            n2921 = disable-structure shown="启用" {
              disable-tunnel: [w1886 w1887] -> w1837
              disable-tunnel: w1835 -> [w1884 w1887]
              frame Disabled {
                n2922 = call <vilib>:"Boolean Crossing PtByPt.vi"("direction"=enum16{"either", "false-true", "true-false"}."true-false", "input"=w1884) -> ("crossing"=w1886:bool)  [unwired: 1 in]
              }
              frame Enabled {
              }
            }
            n2923 = case shown="假" w1837 {
              frame False {
                n2924 = local write "503扫码回复输入"(FALSE ("303扫码回复输入")) -> ()
              }
              frame True {
              }
            }
            n2925 = call <vilib>:"Boolean Crossing PtByPt.vi"("direction"=enum16{"either", "false-true", "true-false"}."false-true", "input"=w1839) -> ("crossing"=w1856:bool)  [unwired: 1 in]
            n2926 = case shown="真" w1856 {
              tunnel: w1858 -> [w2287 w2293]
              tunnel: w1857 -> [w2286 w2292]
              tunnel: [w2286 w2290] -> w1854
              tunnel: [w2287 w2291] -> w1855
              frame False {
              }
              frame True {
                w2294 = u16 0 items=["byte", "word", "Dword"] ("数据类型")
                w2296 = u8 132 items=["I/O (P)"=128, "Input (I)"=129, "Output (Q)"=130, "Bit Memory (M)"=131, "Data (DB)"=132, "Instance Data (DI)"=133, "Local Data (L)"=134, "Predecessor Local Data (VL)"=135] ("寄存器类型")
                n2927 = call "S7_Read.vi"("TCP"=w2293, "DB #"=u16 20, "读取长度"=u16 13, "寄存器类型"=w2296, "起始地址"=u32 60, "数据类型"=w2294, "error in"=w2292) -> ("TCP"=w2291:refnum<k5>, "数据"=w2299:u32[], "error out"=w2301:errorcluster)  [unwired: 5 in, 1 out]
                n2928 = To Unsigned Word Integer(number=w2299) -> (unsigned 16bit integer=w2300:u16[])
                n2929 = call "还原为字符串.vi"("error in (no error)"=w2301, "输入数组"=w2300) -> ("error out"=w2289:errorcluster, "字符串"=w2288:string)  [unwired: 8 in]
                n2930 = stacked-sequence {
                  tunnel: [_ w2305] -> w2290
                  tunnel: w2289 -> [_ w2304]
                  tunnel: w2288 -> [w2302 _]
                  frame #0 {
                    "502二维码" <- w2302
                  }
                  frame #1 {
                    n2931 = property on="ST502扫码请求（事件）" class="Bool (严格)"(error in=w2304, "Val(Sgnl)"=TRUE ("值(信号)")) -> (error out=w2305:errorcluster)  [unwired: 1 in, 1 out]
                  }
                }
              }
            }
            n2932 = disable-structure shown="启用" {
              disable-tunnel: enum16{"either", "false-true", "true-false"}."true-false" ("direction") -> [w1906 _]
              disable-tunnel: [w1905 w1907] -> w1833
              disable-tunnel: w1832 -> [w1904 w1907]
              frame Disabled {
                n2933 = call <vilib>:"Boolean Crossing PtByPt.vi"("direction"=w1906, "input"=w1904) -> ("crossing"=w1905:bool)  [unwired: 1 in]
              }
              frame Enabled {
              }
            }
            n2934 = case shown="假" w1833 {
              frame False {
                n2935 = local write "503数据回复输入"(FALSE ("303数据回复输入")) -> ()
              }
              frame True {
              }
            }
            n2936 = call <vilib>:"Boolean Crossing PtByPt.vi"("direction"=enum16{"either", "false-true", "true-false"}."false-true", "input"=w1836) -> ("crossing"=w1852:bool)  [unwired: 1 in]
            n2937 = case shown="真" w1852 {
              tunnel: w1855 -> [w2167 w2172]
              tunnel: w1854 -> [w2166 w2170]
              tunnel: [w2167 w2220] -> w1846
              tunnel: [w2166 w2182] -> w1845
              frame False {
              }
              frame True {
                w2173 = u16 0 items=["byte", "word", "Dword"] ("数据类型")
                w2175 = u8 132 items=["I/O (P)"=128, "Input (I)"=129, "Output (Q)"=130, "Bit Memory (M)"=131, "Data (DB)"=132, "Instance Data (DI)"=133, "Local Data (L)"=134, "Predecessor Local Data (VL)"=135] ("寄存器类型")
                w2246 = u16 2 items=["byte", "word", "Dword"] ("数据类型")
                w2244 = u8 132 items=["I/O (P)"=128, "Input (I)"=129, "Output (Q)"=130, "Bit Memory (M)"=131, "Data (DB)"=132, "Instance Data (DI)"=133, "Local Data (L)"=134, "Predecessor Local Data (VL)"=135] ("寄存器类型")
                w2252 = u16 1 items=["byte", "word", "Dword"] ("数据类型")
                w2254 = u8 132 items=["I/O (P)"=128, "Input (I)"=129, "Output (Q)"=130, "Bit Memory (M)"=131, "Data (DB)"=132, "Instance Data (DI)"=133, "Local Data (L)"=134, "Predecessor Local Data (VL)"=135] ("寄存器类型")
                w2247 = u16 1 items=["byte", "word", "Dword"] ("数据类型")
                w2249 = u8 132 items=["I/O (P)"=128, "Input (I)"=129, "Output (Q)"=130, "Bit Memory (M)"=131, "Data (DB)"=132, "Instance Data (DI)"=133, "Local Data (L)"=134, "Predecessor Local Data (VL)"=135] ("寄存器类型")
                n2938 = call "S7_Read.vi"("TCP"=w2172, "DB #"=u16 20, "读取长度"=u16 13, "寄存器类型"=w2175, "起始地址"=u32 60, "数据类型"=w2173, "error in"=w2170) -> ("TCP"=w2171:refnum<k5>, "数据"=w2178:u32[], "error out"=w2180:errorcluster)  [unwired: 5 in, 1 out]
                n2939 = To Unsigned Word Integer(number=w2178) -> (unsigned 16bit integer=w2179:u16[])
                n2940 = call "还原为字符串.vi"("error in (no error)"=w2180, "输入数组"=w2179) -> ("error out"=w2169:errorcluster, "字符串"=w2168:string)  [unwired: 8 in]
                n2941 = local write "502二维码"(w2168) -> ()
                n2942 = call "S7_Read.vi"("TCP"=w2171, "DB #"=u16 20, "读取长度"=u16 18, "寄存器类型"=w2244, "起始地址"=u32 140, "数据类型"=w2246, "error in"=w2169) -> ("TCP"=w2237:refnum<k5>, "数据"=w2235:u32[], "error out"=w2236:errorcluster)  [unwired: 5 in, 1 out]
                n2943 = Index Array(array=w2235) -> (element #1=w2241:u32, element #2=w2209:u32, element #3=w2240:u32, element #4=w2239:u32, element #5=w2204:u32, element #6=w2202:u32, element #7=w2234:u32, element #8=w2195:u32, element #9=w2233:u32, element #10=w2232:u32, element #11=w2190:u32, element #12=w2184:u32, element #13=w2231:u32, element #14=w2230:u32, element #15=w2229:u32, element #16=w2228:u32, element #17=w2227:u32, element #18=w2226:u32)  [unwired: 18 in]
                n2944 = Number To Decimal String(number=w2231) -> (decimal integer string=w2217:string)  [unwired: 1 in]
                n2945 = Number To Decimal String(number=w2230) -> (decimal integer string=w2216:string)  [unwired: 1 in]
                n2946 = Number To Decimal String(number=w2229) -> (decimal integer string=w2215:string)  [unwired: 1 in]
                n2947 = Number To Decimal String(number=w2228) -> (decimal integer string=w2214:string)  [unwired: 1 in]
                n2948 = Number To Decimal String(number=w2227) -> (decimal integer string=w2213:string)  [unwired: 1 in]
                n2949 = Number To Decimal String(number=w2226) -> (decimal integer string=w2212:string)  [unwired: 1 in]
                n2950 = Number To Decimal String(number=w2241) -> (decimal integer string=w2225:string)  [unwired: 1 in]
                n2951 = Number To Decimal String(number=w2240) -> (decimal integer string=w2223:string)  [unwired: 1 in]
                n2952 = Number To Decimal String(number=w2239) -> (decimal integer string=w2222:string)  [unwired: 1 in]
                n2953 = Number To Decimal String(number=w2234) -> (decimal integer string=w2221:string)  [unwired: 1 in]
                n2954 = Number To Decimal String(number=w2233) -> (decimal integer string=w2219:string)  [unwired: 1 in]
                n2955 = Number To Decimal String(number=w2232) -> (decimal integer string=w2218:string)  [unwired: 1 in]
                n2956 = Divide(x=w2204, y=u32 100) -> (x/y=w2207:dbl)
                n2957 = Divide(x=w2202, y=u32 100) -> (x/y=w2199:dbl)
                n2958 = Divide(x=w2195, y=u32 100) -> (x/y=w2194:dbl)
                n2959 = Divide(x=w2190, y=u32 100) -> (x/y=w2192:dbl)
                n2960 = Divide(x=w2209, y=u32 100) -> (x/y=w2208:dbl)
                n2961 = Divide(x=w2184, y=u32 100) -> (x/y=w2185:dbl)
                n2962 = Number To Fractional String(number=w2199, precision (6)=i16 2 ("精度(6)")) -> (F-format string=w2198:string)  [unwired: 2 in]
                n2963 = Number To Fractional String(number=w2207, precision (6)=i16 2 ("精度(6)")) -> (F-format string=w2201:string)  [unwired: 2 in]
                n2964 = Number To Fractional String(number=w2194, precision (6)=i16 2 ("精度(6)")) -> (F-format string=w2193:string)  [unwired: 2 in]
                n2965 = Number To Fractional String(number=w2192, precision (6)=i16 2 ("精度(6)")) -> (F-format string=w2189:string)  [unwired: 2 in]
                n2966 = Number To Fractional String(number=w2185, precision (6)=i16 2 ("精度(6)")) -> (F-format string=w2183:string)  [unwired: 2 in]
                n2967 = Number To Fractional String(number=w2208, precision (6)=i16 2 ("精度(6)")) -> (F-format string=w2224:string)  [unwired: 2 in]
                n2968 = call "S7_Read.vi"("TCP"=w2237, "DB #"=u16 20, "读取长度"=u16 1, "寄存器类型"=w2249, "起始地址"=u32 134, "数据类型"=w2247, "error in"=w2236) -> ("TCP"=w2263:refnum<k5>, "数据"=w2265:u32[], "error out"=w2264:errorcluster)  [unwired: 5 in, 1 out]
                n2969 = Index Array(array=w2265) -> (element=w2266:u32)  [unwired: 1 in]
                n2970 = Number To Decimal String(number=w2266) -> (decimal integer string=w2273:string)  [unwired: 1 in]
                n2971 = call "S7_Read.vi"("TCP"=w2263, "DB #"=u16 20, "读取长度"=u16 1, "寄存器类型"=w2254, "起始地址"=u32 126, "数据类型"=w2252, "error in"=w2264) -> ("TCP"=w2220:refnum<k5>, "数据"=w2267:u32[], "error out"=w2211:errorcluster)  [unwired: 5 in, 1 out]
                n2972 = Index Array(array=w2267) -> (element=w2269:u32)  [unwired: 1 in]
                n2973 = Equal?(x=w2269, y=u32 1) -> (x = y?=w2268:bool)
                n2974 = case shown="真" w2268 {
                  tunnel: ["NG" "OK"] -> w2272
                  frame False {
                  }
                  frame True {
                  }
                }
                n2975 = Format Date/Time String(time format string (%c)="%Y-%m-%d" ("时间格式字符串(%c)")) -> (date/time string=w2270:string)  [unwired: 2 in]
                n2976 = Get Date/Time String(want seconds? (F)=TRUE ("需要秒？(F)")) -> (time string=w2271:string)  [unwired: 2 in, 1 out]
                n2977 = Insert Into Array(array=string[] [] ("数组"), index=0 ("索引"), new element #1="502" ("新元素/子数组"), new element #2=w2272, new element #3=w2270, new element #4=w2271, new element #5=w2272, new element #6=w2273, new element #7=w2225, new element #8=w2224, new element #9=w2223, new element #10=w2222, new element #11=w2201, new element #12=w2198, new element #13=w2221, new element #14=w2193, new element #15=w2219, new element #16=w2218, new element #17=w2189, new element #18=w2183, new element #19=w2217, new element #20=w2216, new element #21=w2215, new element #22=w2214, new element #23=w2213, new element #24=w2212) -> (w2181:string[])
                n2978 = stacked-sequence {
                  seq-local: [w2275 _] -> [_ w2279]
                  tunnel: w2211 -> [w2275 _]
                  tunnel: [_ w2276] -> w2182
                  tunnel: w2181 -> [w2274 _]
                  frame #0 {
                    "502数据" <- w2274
                  }
                  frame #1 {
                    n2979 = property on="ST502数据读取（事件）" class="Bool (严格)"(error in=w2279, "Val(Sgnl)"=TRUE ("值(信号)")) -> (error out=w2277:errorcluster)  [unwired: 1 in, 1 out]
                    n2980 = disable-structure shown="禁用" {
                      disable-tunnel: w2277 -> [w2281 w2283]
                      disable-tunnel: [w2280 w2283] -> w2276
                      frame Disabled {
                        n2981 = property on="ST502画曲线" class="Bool (严格)"(error in=w2281, "Val(Sgnl)"=TRUE ("值(信号)")) -> (error out=w2280:errorcluster)  [unwired: 1 in, 1 out]
                      }
                      frame Enabled {
                      }
                    }
                  }
                }
              }
            }
            n2982 = call <vilib>:"Boolean Crossing PtByPt.vi"("direction"=enum16{"either", "false-true", "true-false"}."false-true", "input"=w1835) -> ("crossing"=w1848:bool)  [unwired: 1 in]
            n2983 = case shown="真" w1848 {
              tunnel: w1846 -> [w2147 w2153]
              tunnel: w1845 -> [w2146 w2152]
              tunnel: [w2146 w2149] -> w1841
              tunnel: [w2147 w2151] -> w1842
              frame False {
              }
              frame True {
                w2154 = u16 0 items=["byte", "word", "Dword"] ("数据类型")
                w2156 = u8 132 items=["I/O (P)"=128, "Input (I)"=129, "Output (Q)"=130, "Bit Memory (M)"=131, "Data (DB)"=132, "Instance Data (DI)"=133, "Local Data (L)"=134, "Predecessor Local Data (VL)"=135] ("寄存器类型")
                n2984 = call "S7_Read.vi"("TCP"=w2153, "DB #"=u16 20, "读取长度"=u16 13, "寄存器类型"=w2156, "起始地址"=u32 82, "数据类型"=w2154, "error in"=w2152) -> ("TCP"=w2151:refnum<k5>, "数据"=w2159:u32[], "error out"=w2161:errorcluster)  [unwired: 5 in, 1 out]
                n2985 = To Unsigned Word Integer(number=w2159) -> (unsigned 16bit integer=w2160:u16[])
                n2986 = call "还原为字符串.vi"("error in (no error)"=w2161, "输入数组"=w2160) -> ("error out"=w2150:errorcluster, "字符串"=w2148:string)  [unwired: 8 in]
                n2987 = stacked-sequence {
                  tunnel: w2150 -> [_ w2165]
                  tunnel: [_ w2164] -> w2149
                  tunnel: w2148 -> [w2162 _]
                  frame #0 {
                    "503二维码" <- w2162
                  }
                  frame #1 {
                    n2988 = property on="ST503扫码请求（事件）" class="Bool (严格)"(error in=w2165, "Val(Sgnl)"=TRUE ("值(信号)")) -> (error out=w2164:errorcluster)  [unwired: 1 in, 1 out]
                  }
                }
              }
            }
            n2989 = call <vilib>:"Boolean Crossing PtByPt.vi"("direction"=enum16{"either", "false-true", "true-false"}."false-true", "input"=w1832) -> ("crossing"=w1843:bool)  [unwired: 1 in]
            n2990 = case shown="真" w1843 {
              tunnel: w1842 -> [w2075 w2079]
              tunnel: w1841 -> [w2074 w2078]
              tunnel: [w2075 w2108] -> w1829
              tunnel: [w2074 w2090] -> w1828
              frame False {
              }
              frame True {
                w2081 = u16 0 items=["byte", "word", "Dword"] ("数据类型")
                w2083 = u8 132 items=["I/O (P)"=128, "Input (I)"=129, "Output (Q)"=130, "Bit Memory (M)"=131, "Data (DB)"=132, "Instance Data (DI)"=133, "Local Data (L)"=134, "Predecessor Local Data (VL)"=135] ("寄存器类型")
                w2107 = u16 1 items=["byte", "word", "Dword"] ("数据类型")
                w2105 = u8 132 items=["I/O (P)"=128, "Input (I)"=129, "Output (Q)"=130, "Bit Memory (M)"=131, "Data (DB)"=132, "Instance Data (DI)"=133, "Local Data (L)"=134, "Predecessor Local Data (VL)"=135] ("寄存器类型")
                w2114 = u16 1 items=["byte", "word", "Dword"] ("数据类型")
                w2116 = u8 132 items=["I/O (P)"=128, "Input (I)"=129, "Output (Q)"=130, "Bit Memory (M)"=131, "Data (DB)"=132, "Instance Data (DI)"=133, "Local Data (L)"=134, "Predecessor Local Data (VL)"=135] ("寄存器类型")
                w2109 = u16 1 items=["byte", "word", "Dword"] ("数据类型")
                w2111 = u8 132 items=["I/O (P)"=128, "Input (I)"=129, "Output (Q)"=130, "Bit Memory (M)"=131, "Data (DB)"=132, "Instance Data (DI)"=133, "Local Data (L)"=134, "Predecessor Local Data (VL)"=135] ("寄存器类型")
